vi "writeCSV(Multi-Line).vi"(8 "error in (no error)":errorcluster, 9 "Array":dbl[][](array[numeric]), 10 "file path (use dialog)":path=path "C:/Users/RoboIme/git/sslview/Util/Farias2.csv", 11 "Utilities in":refnum<class "Utilities.lvclass">) -> (0 "error out":errorcluster, 3 "Utilities out":refnum<class "Utilities.lvclass">)   [LabVIEW 2023, in "Utilities.lvclass"]
uses:
  Utilities.lvclass
panel:
  out "refnum out":refnum<file>
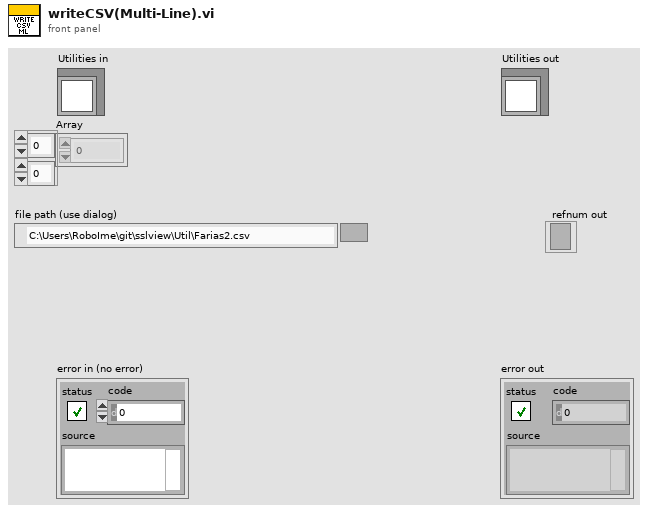
[diagram p1: front panel]
types:
  T1 = enum16{"open", "replace", "create", "open or create", "replace or create", "replace or create with confirmation"}
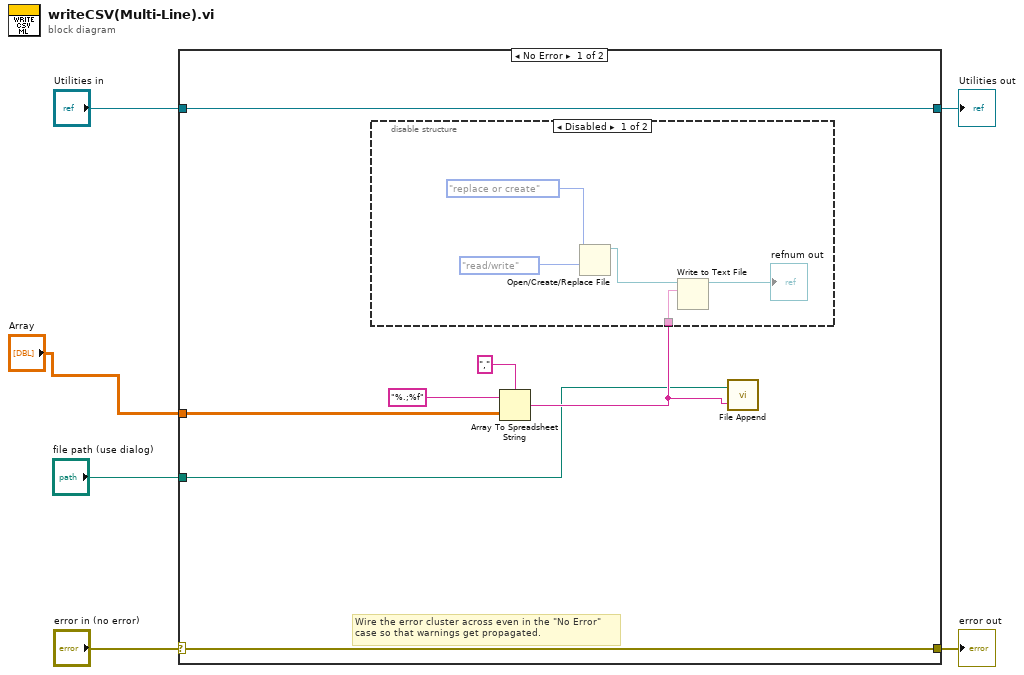
[diagram p0: block diagram]
diagram:
  n1 = case shown="No Error" "error in (no error)" {
    selector: "error in (no error)" -> [w12 w20]
    tunnel: [w12 w20] -> w5
    tunnel: [w13 w19] -> w3
    tunnel: "Utilities in" -> [w13 w19]
    tunnel: "Array" -> [w8 _]
    tunnel: "file path (use dialog)" -> [w7 _]
    frame No Error {
      # "Wire the error cluster across even in the \"No Error\"\ncase so that warnings get propagated."
      n2 = Array To Spreadsheet String(delimiter (Tab)=",", array=w8, 3:"%.;%f" ("format string")) -> (spreadsheet string=w9:string)
      n3 = disable-structure shown="Disabled" {
        disable-tunnel: w9 -> [w18 _]
        frame Disabled {
          n4 = Open/Create/Replace File(operation (0:open)=T1."replace or create", access (0:read/write)=enum16{"read/write", "read-only", "write-only"}."read/write") -> (refnum out=w15:refnum<file>)  [unwired: 4 in, 2 out]
          n5 = Write to Text File(file (use dialog)=w15, text=w18) -> (refnum out=→"refnum out":refnum<file>)  [unwired: 2 in, 2 out]
        }
        frame Enabled {
        }
      }
      n6 = call "File Append.vi"("string"=w9, "file path"=w7) -> ()  [unwired: 2 in]
    }
    frame Error {
    }
  }
  "error out" <- w5
  "Utilities out" <- w3
